vi "[RT]Main.vi"() -> ()   [LabVIEW 2018]
doc: "The myRIO Project template acquires acceleration data from the onboard accelerometer and displays the changes of acceleration values in a waveform chart."
uses:
  TypeDef/ControllerState.ctl
  TypeDef/CMD Cluster.ctl
  <vilib>/myRIO/Common/Instrument Driver Framework/myRIO v1.0/UART/vis/myRIO v1.0 Close UART.vi
  [GlobVar]SensorState.vi
  <vilib>/myRIO/Common/Instrument Driver Framework/Utilities/vis/FPGA Ref Manager.vi
  <vilib>/myRIO/Common/Instrument Driver Framework/myRIO v1.0/myRIO v1.0 Reset FPGA.vi
  <vilib>/myRIO/Common/Instrument Driver Framework/myRIO v1.0/IRQ/vis/myRIO v1.0 IRQ Info FGV.vi
  <vilib>/myRIO/Common/Instrument Driver Framework/myRIO v1.0/IRQ/vis/myRIO v1.0 Timer IRQ Info FGV.vi
  <vilib>/myRIO/Common/Instrument Driver Framework/myRIO v1.0/IRQ/vis/myRIO v1.0 ISR Agent.vi
  <vilib>/myRIO/Instrument Drivers/Utilities/Utilities.lvlib
panel:
  out "error out":errorcluster
  in  "Stop":bool
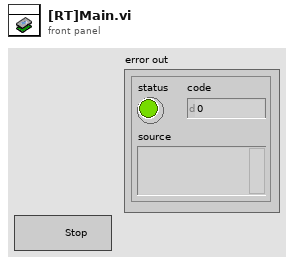
[diagram p1: front panel]
types:
  T1 = typedef "CMD Cluster.ctl" = cluster{"timestamp":u32, "State Rqst":T2, "target-temp":dbl, "target-volume":dbl}
  T2 = typedef "ControllerState.ctl" = enum16{"Idle", "Vorheizen", "Brühen", "Emergency-Stop"}
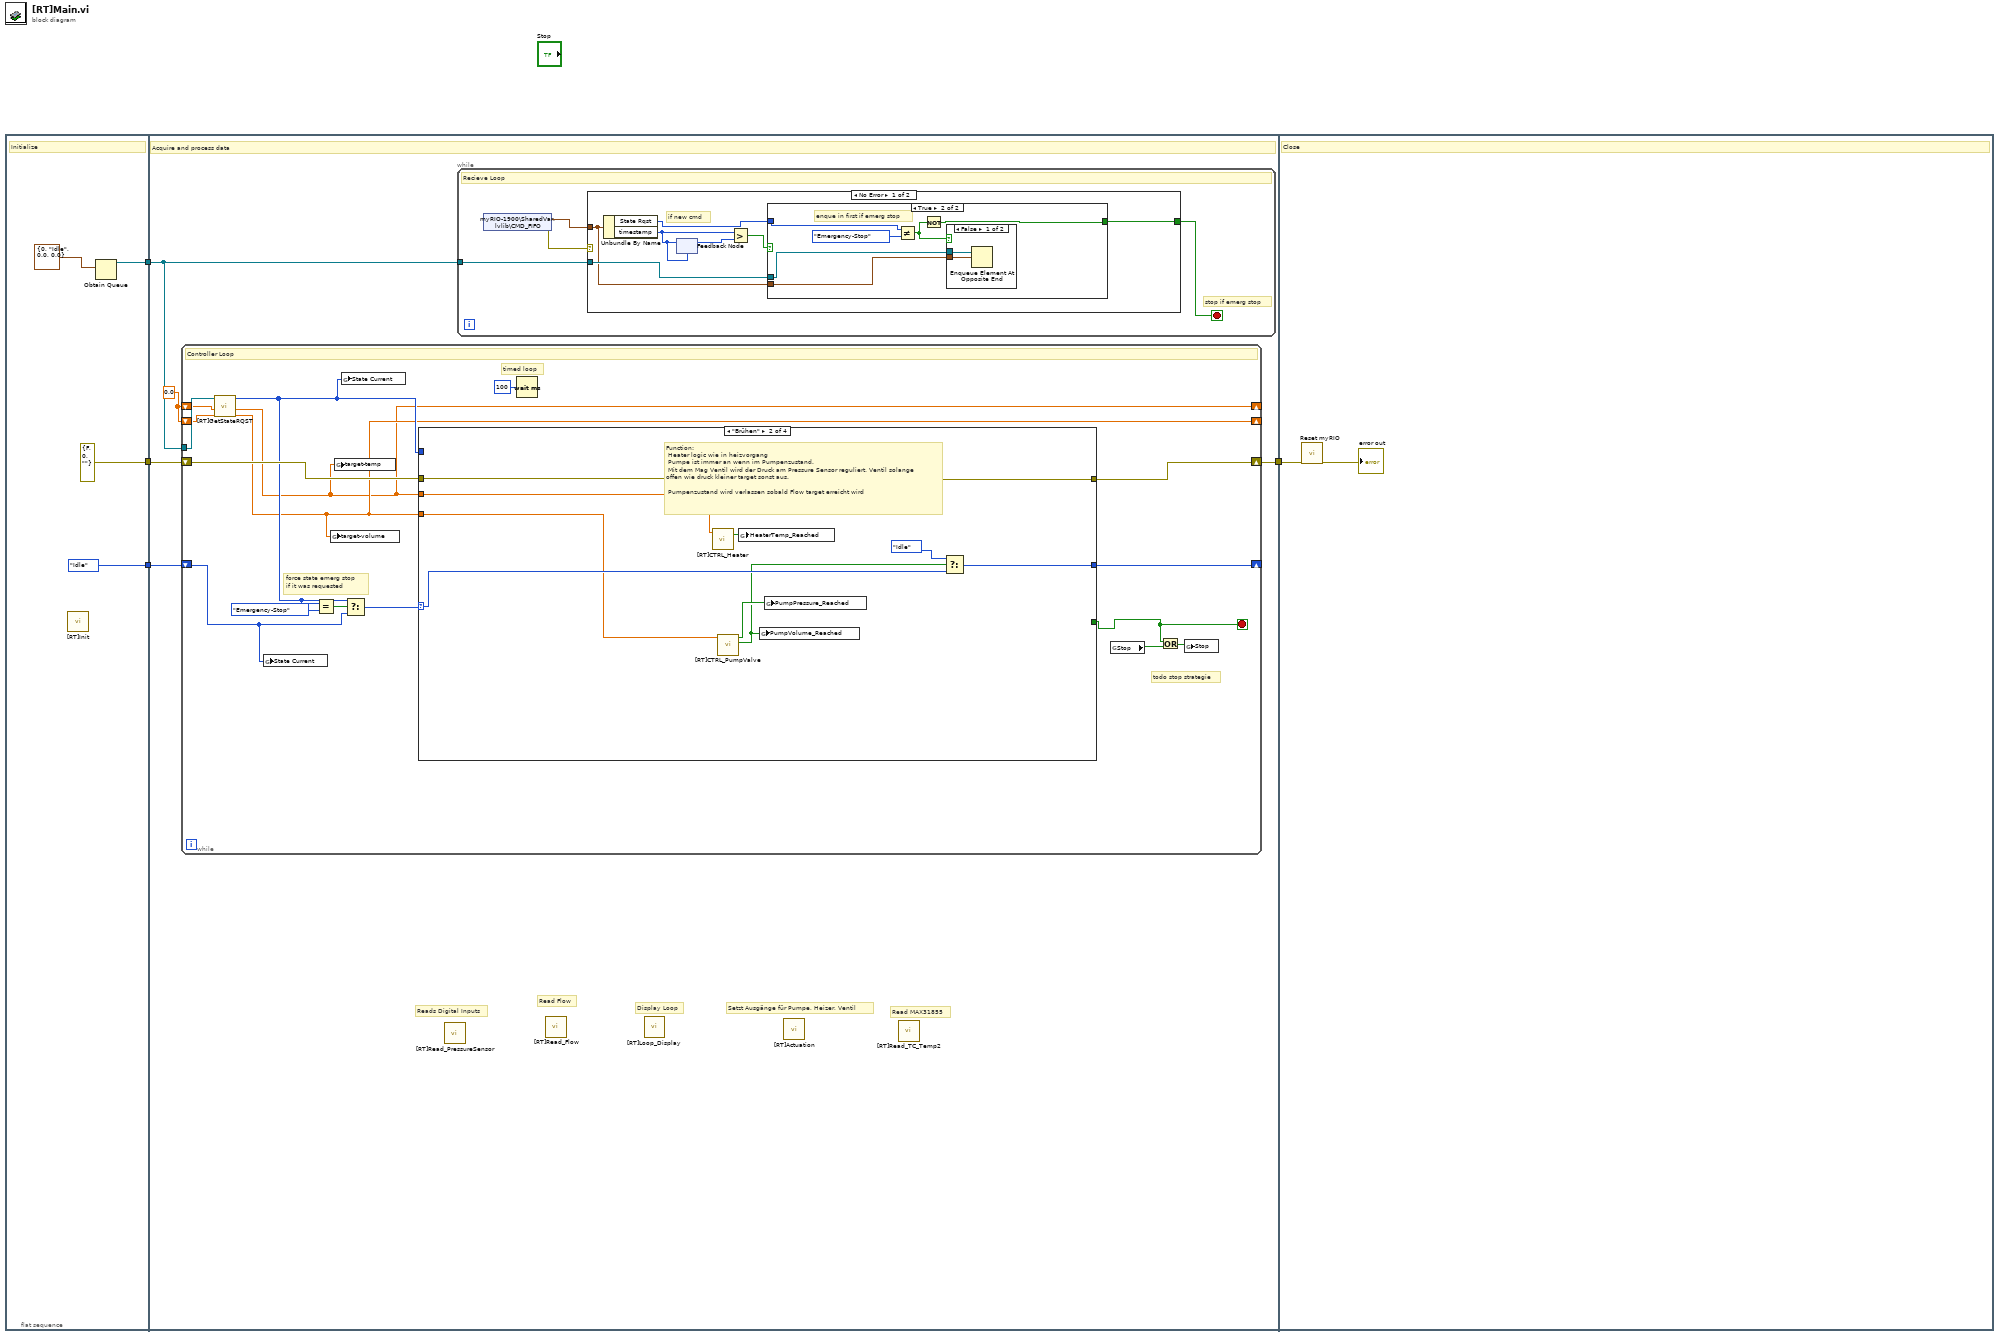
[diagram p0: block diagram]
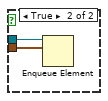
[diagram p3: hidden frame]
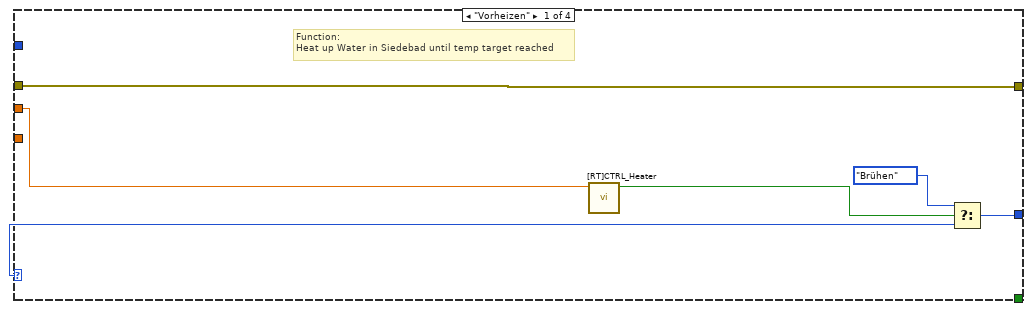
[diagram p5: hidden frame]
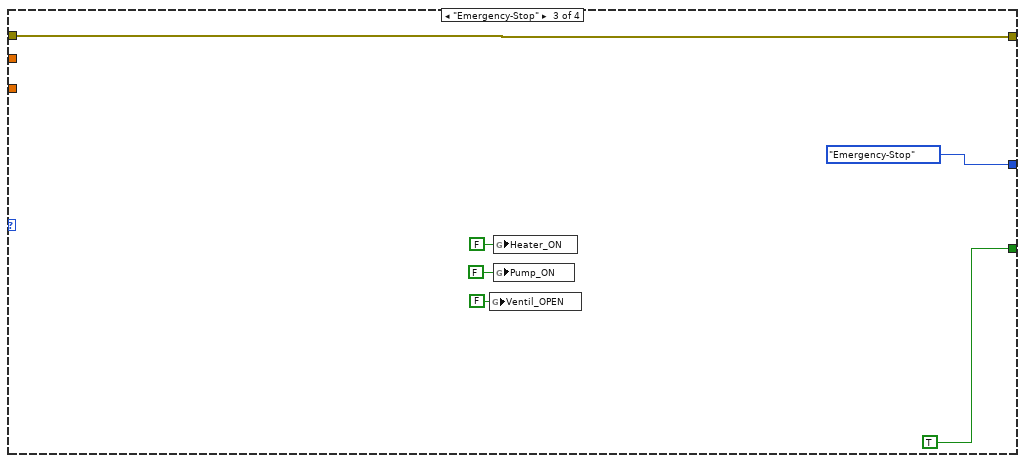
[diagram p6: hidden frame]
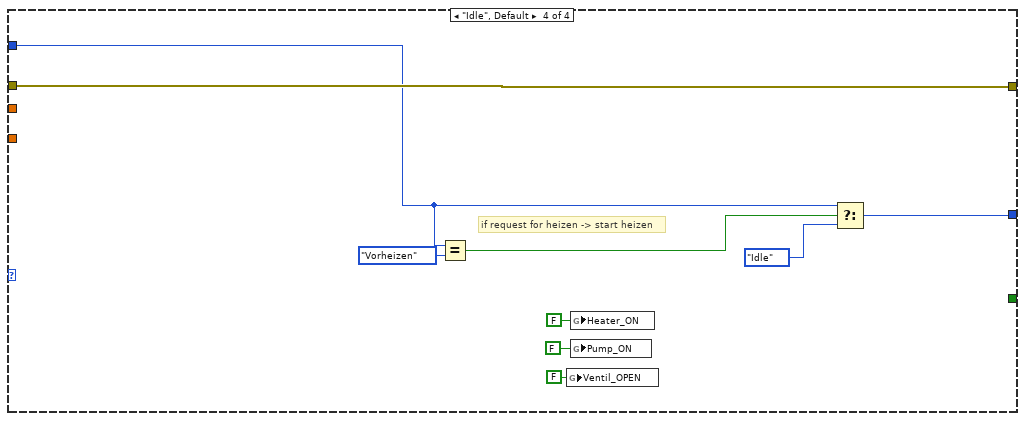
[diagram p7: hidden frame]
diagram:
  n1 = flat-sequence {
    tunnel: [errorcluster {"status"=FALSE, "code"=0, "source"=""} ("error in (no error)")] -> w4
    tunnel: [ControllerState."Idle"] -> w2
    tunnel: [w5] -> w1
    tunnel: w4 -> [w13]
    tunnel: [w12] -> w3
    tunnel: w2 -> [w11]
    tunnel: w1 -> [w10]
    tunnel: w3 -> [w83]
    frame #0 {
      # "Initialize"
      n2 = call "[RT]Init.vi"() -> ()  [unwired: 12 in]
      n3 = Obtain Queue(element data type=T1 {"timestamp"=0, "State Rqst"=enum."Idle", "target-temp"=0.0, "target-volume"=0.0} ("CMD Cluster")) -> (queue out=w5:refnum<queue>)  [unwired: 4 in, 2 out]
    }
    frame #1 {
      w9 = 0.0 ("target-volume")
      # "Read Flow"
      # "Read MAX31855"
      # "Display Loop"
      # "Reads Digital Inputs"
      # "Setzt Ausgänge für Pumpe, Heizer, Ventil"
      # "Acquire and process data"
      n4 = while {
        shift-right: [w50] -> w12
        shift-left: w13 -> [w51]
        shift-right: [w49] -> _
        shift-left: w11 -> [w38]
        tunnel: w10 -> [w48]
        shift-right: [w36] -> _
        shift-left: w9 -> [w39]
        shift-right: [w35] -> _
        shift-left: w9 -> [w40]
        stop <- w41 stop-if-true
        # "todo stop strategie"
        # "force state emerg stop \nif it was requested"
        # "timed loop"
        # "Controller Loop"
        n5 = call "[RT]GetStateRQST.vi"("target-volume out"=w39, "target-temp in"=w40, "Queue in"=w48) -> ("target-volume"=w36:dbl, "target-temp"=w35:dbl, "State Rqst"=w37:T2)  [unwired: 6 in]
        n6 = global write "[GlobVar]SensorState.vi" "State Current"(w38) -> ()
        n7 = Equal?(x=w37, y=ControllerState."Emergency-Stop") -> (x = y?=w46:bool)
        n8 = global write "[GlobVar]SensorState.vi" "target-volume"(w36) -> ()
        n9 = global write "[GlobVar]SensorState.vi" "target-temp"(w35) -> ()
        n10 = global write "[GlobVar]SensorState.vi" "State Current"(w37) -> ()
        n11 = Select(t=w37, s=w46, f=w38) -> (s? t:f=w44:T2)
        n12 = case shown="\"Brühen\"" w44 {
          selector: w44 -> [w55 w63 _ _]
          tunnel: w51 -> [w57 w66 w72 w81]
          tunnel: [w57 w66 w72 w81] -> w50
          tunnel: [_ _ TRUE _] -> w41
          tunnel: [w56 w65 ControllerState."Emergency-Stop" w80] -> w49
          tunnel: w37 -> [_ _ _ w76]
          tunnel: w35 -> [w53 w62 _ _]
          tunnel: w36 -> [_ w58 _ _]
          frame "Vorheizen" {
            # "Function: \nHeat up Water in Siedebad until temp target reached"
            n13 = call "[RT]CTRL_Heater.vi"("target-temp"=w53) -> ("temp_reached"=w52:bool)  [unwired: 10 in]
            n14 = Select(t=ControllerState."Brühen", s=w52, f=w55) -> (s? t:f=w56:T2)
          }
          frame "Brühen" {
            # "Function:\n\tHeater logic wie in heizvorgang\n\tPumpe ist immer an wenn im Pumpenzustand.\n\tMit dem Mag Ventil wird der Druck am Pressure Sensor reguliert. Ventil solange offen wie druck kleiner target sonst aus.\n\t\n\tPumpenzustand wird verlassen sobald Flow target erreicht wird"
            n15 = call "[RT]CTRL_Heater.vi"("target-temp"=w62) -> ("temp_reached"=w61:bool)  [unwired: 10 in]
            n16 = call "[RT]CTRL_PumpValve.vi"("target-volume"=w58) -> ("volume reached"=w59:bool, "pressure reached"=w60:bool)  [unwired: 9 in]
            n17 = global write "[GlobVar]SensorState.vi" "HeaterTemp_Reached"(w61) -> ()
            n18 = global write "[GlobVar]SensorState.vi" "PumpVolume_Reached"(w59) -> ()
            n19 = global write "[GlobVar]SensorState.vi" "PumpPressure_Reached"(w60) -> ()
            n20 = Select(t=ControllerState."Idle", s=w59, f=w63) -> (s? t:f=w65:T2)
          }
          frame "Emergency-Stop" {
            n21 = global write "[GlobVar]SensorState.vi" "Ventil_OPEN"(FALSE ("Heater_ON")) -> ()
            n22 = global write "[GlobVar]SensorState.vi" "Heater_ON"(FALSE ("Heater_ON")) -> ()
            n23 = global write "[GlobVar]SensorState.vi" "Pump_ON"(FALSE ("Heater_ON")) -> ()
          }
          frame "Idle", Default {
            # "if request for heizen -> start heizen"
            n24 = Equal?(x=w76, y=ControllerState."Vorheizen") -> (x = y?=w77:bool)
            n25 = global write "[GlobVar]SensorState.vi" "Ventil_OPEN"(FALSE ("Heater_ON")) -> ()
            n26 = global write "[GlobVar]SensorState.vi" "Heater_ON"(FALSE ("Heater_ON")) -> ()
            n27 = global write "[GlobVar]SensorState.vi" "Pump_ON"(FALSE ("Heater_ON")) -> ()
            n28 = Select(t=w76, s=w77, f=ControllerState."Idle") -> (s? t:f=w80:T2)
          }
        }
        n29 = Wait (ms)(milliseconds to wait=u32 100) -> ()  [unwired: 1 out]
        n30 = global read "[GlobVar]SensorState.vi" "Stop"() -> (w43:bool)
        n31 = Or(x=w41, y=w43) -> (x .or. y?=w42:bool)
        n32 = global write "[GlobVar]SensorState.vi" "Stop"(w42) -> ()
      }
      n33 = call "[RT]Read_PressureSensor.vi"() -> ()  [unwired: 11 in]
      n34 = while {
        tunnel: w10 -> [w17]
        stop <- w14 stop-if-true
        # "stop if emerg stop"
        # "Recieve Loop"
        n35 = shared-variable "myRIO-1900\\SharedVar.lvlib\\CMD_FIFO"() -> (w16:T1, error out=w15:errorcluster)  [unwired: 1 in]
        n36 = case shown="No Error" w15 {
          tunnel: w17 -> [w22 _]
          tunnel: w16 -> [w21 _]
          tunnel: [w19 _] -> w14
          frame No Error {
            # "if new cmd"
            n37 = Unbundle By Name(w21) -> ("State Rqst"=w20:T2, "timestamp"=w18:u32)
            n38 = feedback #1(w18) -> (w24:u32)
            n39 = feedback-in #1(w18) -> ()
            n40 = Greater?(x=w18, y=w24) -> (0:w23:bool)
            n41 = case shown="True" w23 {
              tunnel: w22 -> [_ w30]
              tunnel: w21 -> [_ w29]
              tunnel: w20 -> [_ w28]
              tunnel: [_ w25] -> w19
              frame False {
              }
              frame True {
                # "enque in first if emerg stop"
                n42 = Not Equal?(x=w28, y=ControllerState."Emergency-Stop") -> (x != y?=w26:bool)
                n43 = Not(x=w26) -> (.not. x?=w25:bool)
                n44 = case shown="False" w26 {
                  tunnel: w30 -> [w31 w34]
                  tunnel: w29 -> [w32 w33]
                  frame False {
                    n45 = Enqueue Element At Opposite End(queue=w31, element=w32) -> ()  [unwired: 2 in, 3 out]
                  }
                  frame True {
                    n46 = Enqueue Element(queue=w34, element=w33) -> ()  [unwired: 2 in, 3 out]
                  }
                }
              }
            }
          }
          frame Error {
          }
        }
      }
      n47 = call "[RT]Read_Flow.vi"() -> ()  [unwired: 9 in, 2 out]
      n48 = call "[RT]Loop_Display.vi"() -> ()  [unwired: 12 in]
      n49 = call "[RT]Actuation.vi"() -> ()  [unwired: 12 in]
      n50 = call "[RT]Read_TC_Temp2.vi"() -> ()  [unwired: 10 in, 2 out]
    }
    frame #2 {
      # "Close"
      n51 = call <vilib>:"Reset myRIO.vi"("error in (no error)"=w83) -> ("error out"=→"error out":errorcluster)  [unwired: 10 in]
    }
  }
